vi "ma_Check Segmented Limit (array X Y).vi"(0 "Specification Cluster":cluster{"X":dbl[], "Y":dbl[]}[](array[cluster]) {"Y" format="%0.2f"; "X" format="%0.2f"}, 1 "x0":dbl format="%0.2f", 2 "dx":dbl format="%0.2f", 3 "error in":errorcluster) -> (8 "limit spec ok":bool, 9 "1st valid segment index":i32, 10 "error out":errorcluster)   [LabVIEW 2020, in "NI_MAPro.lvlib"]
uses:
  NI_MAPro.lvlib
  NI_MABase.lvlib
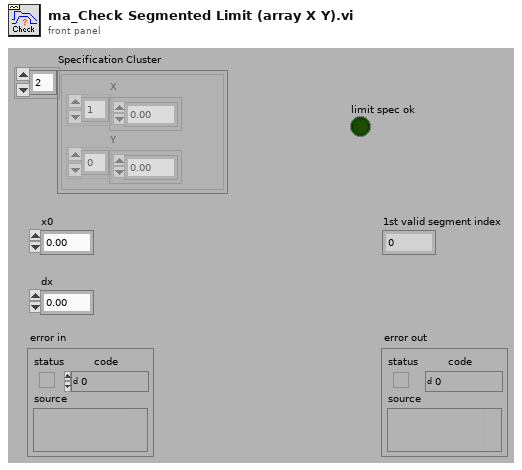
[diagram p1: front panel]
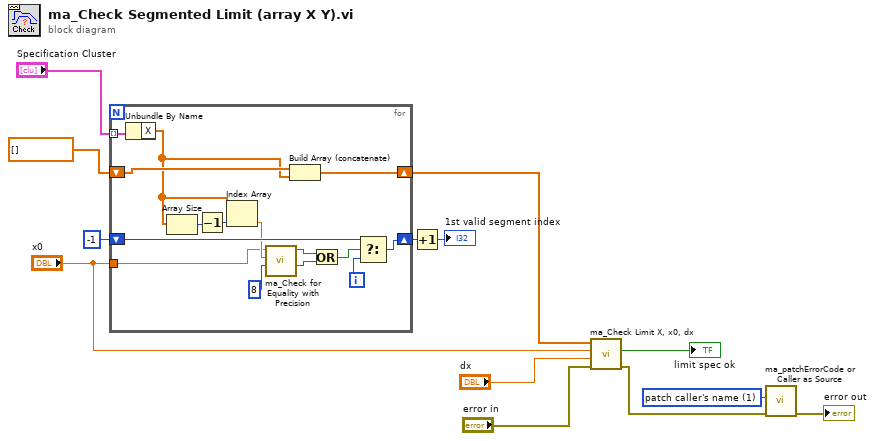
[diagram p0: block diagram]
diagram:
  w3 = u16 1 items=["patch error code", "patch caller's name"] ("operation")
  n1 = for {
    tunnel: "Specification Cluster" -> [w28] mode=indexing
    shift-right: [w14] -> w9
    shift-left: dbl[] [] ("element") -> [w27]
    shift-right: [w23] -> w5
    shift-left: -1 -> [w24]
    tunnel: "x0" -> [w19]
    i -> [w21]
    n2 = Unbundle By Name(w28) -> ("X"=w22:dbl[])
    n3 = Array Size(array=w22) -> (size(s)=w26:i32)
    n4 = Decrement(x=w26) -> (x-1=w25:i32)
    n5 = Index Array(array=w22, index=w25) -> (element=w20:dbl)
    n6 = call "ma_Check for Equality with Precision.vi"("precision"=8, "n2"=w20, "n1"=w19) -> ("n1 < n2?"=w16:bool, "equal (within precision)"=w17:bool)  [unwired: 7 out]
    n7 = Build Array (concatenate)(w27, w22) -> (w14:dbl[])
    n8 = Or(x=w17, y=w16) -> (x .or. y?=w15:bool)
    n9 = Select(t=w24, s=w15, f=w21) -> (s? t:f=w23:i32)
  }
  n10 = Increment(x=w5) -> (x+1=→"1st valid segment index":i32)
  n11 = call "ma_Check Limit X, x0, dx.vi"("X"=w9, "x0"="x0", "dx"="dx", "error in"="error in") -> ("limit spec ok"=→"limit spec ok":bool, "error out"=w2:errorcluster)  [unwired: 5 out]
  n12 = call "ma_patchErrorCode or Caller as Source.vi"("error in (no error)"=w2, "operation"=w3) -> ("error out"=→"error out":errorcluster)  [unwired: 2 in, 7 out]
